vi "FillSurfaceRect.vi"(7 "Entire Surface (F)":bool, 8 "No Error":errorcluster, 9 "Color":u32, 10 "Rect":T1, 11 "Dst [SDL_Surface *]":T2 format="%.0x") -> (0 "error out":errorcluster)   [LabVIEW 2026, in "SDL3.lvlib" / "Surface.lvlib"]
doc: "<B>Summary</B>\nPerform a fast fill of a rectangle with a specific color.\n\n<B>Remarks</B>\ncolor should be a pixel of the format used by the surface, and can be generated by SDL_MapRGB() or SDL_MapRGBA(). If the color value contains an alpha component then the destination is simply filled with that alpha information, no blending takes place.\n\nIf there is a clip rectangle set on the destination (set via SDL_SetSurfaceClipRect()), then this function will fill based on the intersection of the clip rectangle and rect."
uses:
  Surface.lvlib
  Rect/Rect--cluster.ctl
  <vilib>/Utility/error.llb/Error Cluster From Error Code.vi
  Error/Error.lvlib
  Lib/SDL3.dll
  Rect/Rect.lvlib
  SDL_Surface--pointer.ctl
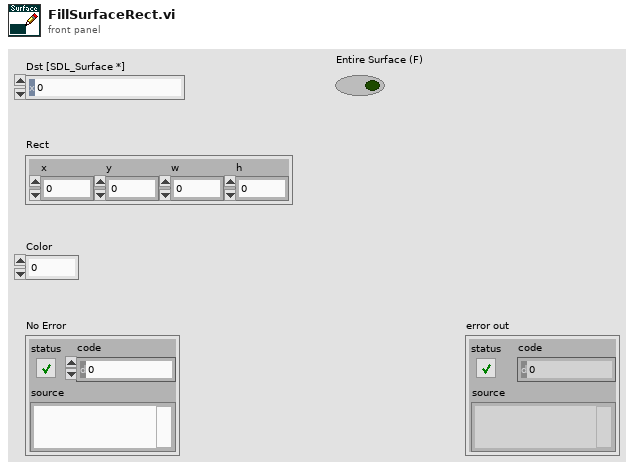
[diagram p1: front panel]
types:
  T1 = typedef "SDL3.lvlib/Rect.lvlib/Rect--cluster.ctl" = cluster{"x":i32, "y":i32, "w":i32, "h":i32}
  T2 = typedef "SDL3.lvlib/Surface.lvlib/SDL_Surface--pointer.ctl" = i64
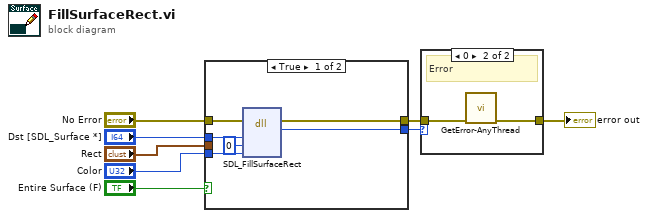
[diagram p0: block diagram]
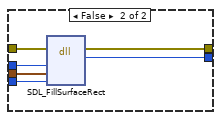
[diagram p2: hidden frame]
diagram:
  n1 = case shown="True" "Entire Surface (F)" {
    tunnel: "No Error" -> [w14 w20]
    tunnel: [w13 w19] -> w2
    tunnel: [w12 w18] -> w1
    tunnel: "Dst [SDL_Surface *]" -> [w11 w17]
    tunnel: "Rect" -> [_ w16]
    tunnel: "Color" -> [w10 w15]
    frame True {
      n2 = dll-call lib="C:/Users/saukko/Dev/LV-SDL3/Sources/SDL3/Lib/SDL3.*" fn="SDL_FillSurfaceRect"(error in=w14, "dst"=w11, "rect"=i64 0, "color"=w10) -> (error out=w13:errorcluster, "return type"=w12:i32)  [unwired: 5 in, 1 out]
    }
    frame False {
      n3 = dll-call lib="C:/Users/saukko/Dev/LV-SDL3/Sources/SDL3/Lib/SDL3.*" fn="SDL_FillSurfaceRect"(error in=w20, "dst"=w17, "rect"=w16, "color"=w15) -> (error out=w19:errorcluster, "return type"=w18:i32)  [unwired: 5 in, 1 out]
    }
  }
  n4 = case shown="0" w1 {
    tunnel: w2 -> [w21 w23]
    tunnel: [w21 w22] -> w7
    frame Default {
      # "Ok"
    }
    frame 0 {
      # "Error"
      n5 = call "GetError-AnyThread.vi"("No Error"=w23) -> ("Error Out"=w22:errorcluster)  [unwired: 10 in]
    }
  }
  "error out" <- w7
